vi "Square Root.vi"   [LabVIEW 2010, in "NI_Matrix.lvlib"]
doc: "Computes the square root of the input matrix."
uses:
  NI_Matrix.lvlib
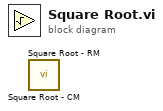
[diagram p0: block diagram]
diagram:
  n1 = call "Square Root - CM.vi"() -> ()  [unwired: 1 in, 1 out]
  n2 = call "Square Root - RM.vi"() -> ()  [unwired: 1 in, 1 out]
